vi "201786.vi"() -> ()   [LabVIEW 2013]
doc: "This simple example demonstrates the use of the relative time axis, synchronized with the system clock. This example uses the Timed Loop structure to determine the loop timing as well as the delta X for the points on the strip-chart. \n\nUsing the Timed Loop, along with the correct setting of two of its properties, ensures the accuracy of the time values displayed on the bottom of the chart. Double-click the Input Node of the Timed Loop, to observe the Discard missed periods option is not checked and the Maintain original phase option is checked. If you control timing using the Wait Until Next ms Multiple function, as demonstrated in the example program entitled \"Real-Time Chart\" (refer to the Developer Zone for this example), jitter causes delays in the execution of the While Loop. Over time, these delays complie and the time values displayed at the bottom of the chart drifts from the actual system clock. By using the Timed Loop, you can compensate for unexpected delays in subsequent iterations of the loop. This ensures the time values displayed on the bottom of the chart stay synchronized with the system clock.\n\nYou can use this example as a prototype for applications that acquire data at a constant, known rate. You determine the maximum rate using the timer resolution and speed of your machine. \n\nNote: The Period of Loop (ms) input in this example allows a minimum of 50 ms. This prevents the user from attempting to set the period to less than the actual time needed to execute the iteration. You can change this minimum value by changing the properties of the Period of Loop (ms) input.\n\nNote the use of Unbundle by Name function to extract the current time information, as well as the use of the Chart Property Node to set the X axis as desired. The current example displays 10 seconds of data regardless of the sample rate determined by the Period of Loop (ms) input."
uses:
  <vilib>/Platform/TimedLoop/XDataNode/timing_clust.ctl
  <vilib>/Platform/TimedLoop/XDataNode/nitl_modes.ctl
  <vilib>/Platform/TimedLoop/XDataNode/wakeup.ctl
  <vilib>/platform/TimedLoop/XDataNode/XDataNode.xnode
  <vilib>/Platform/TimedLoop/XDataNode/XDNodeRunTimeDep.lvlib
panel:
  in  "stop":bool
  out "Strip Chart":cluster{dbl, dbl}(graph)={0.6048539044559809, 0.9356575577636529}
  in  "Period of Loop (ms)":u32(knob)=50 min=50 scale=0.0..2000.0
  # "Select Help»Show Context Help and move the cursor\nover the VI icon to display help for this VI."
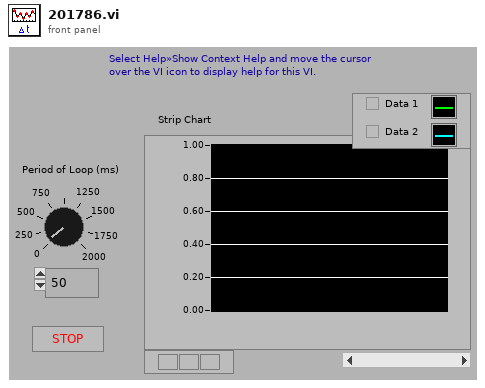
[diagram p1: front panel]
types:
  T1 = cluster{"second":i32, "minute":i32, "hour":i32, "day of month":i32, "month":i32, "year":i32, "day of week":i32, "day of year":i32, "is DST":i32}
  T2 = typedef "XDNodeRunTimeDep.lvlib/timing_clust.ctl" = cluster{"Expected End [f-1]":u64, "Actual End [f-1]":u64, "Finished Late? [f-1]":bool, "Expected End [i-1]":u64, "Actual End [i-1]":u64, "Finished Late? [i-1]":bool, "Expected Start [i]":u64, "Actual Start [i]":u64, "Expected Start [f]":u64, "Actual Start [f]":u64, "Source Name":string, "Structure Name":string, "Period":i64, "Deadline":i64, "Offset":i64, "Start":i64, "Priority":i32, "Timeout":i32, "Mode":T3, "Wakeup Reason":T4, "Error":errorcluster, "Source Type":string, "Secondary Source Type":string, "Global End Time":u64, "Global Start Time":u64, "Frame Duration":u64, "Iteration Duration":u64, "Assigned CPU":i32, "I/O Scan Engine Mode":u32}
  T3 = typedef "XDNodeRunTimeDep.lvlib/nitl_modes.ctl" = enum32{"No Change", "Process missed periods, maintain original phase", "Discard missed periods, maintain original phase", "Process missed periods, ignore original phase", "Discard missed periods, ignore original phase"}
  T4 = typedef "XDNodeRunTimeDep.lvlib/wakeup.ctl" = enum32{"Normal", "Aborted", "Asynchronous wakeup", "Timing source error", "Timed loop error", "Timeout"}
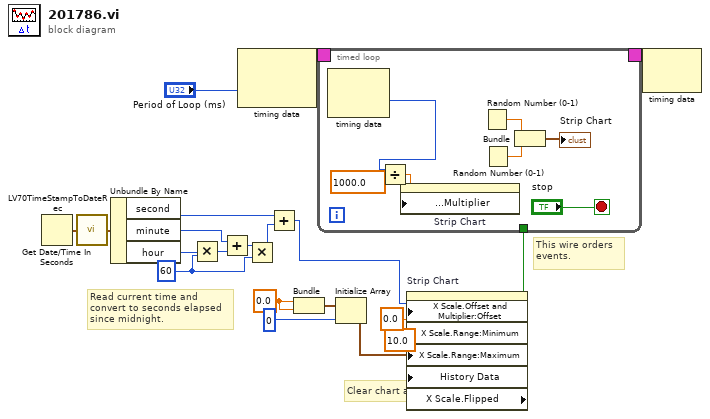
[diagram p0: block diagram]
diagram:
  w9 = 0.0
  w13 = 60
  # "This wire orders\nevents."
  # "Clear chart and set the X axis."
  # "Read current time and\nconvert to seconds elapsed\nsince midnight."
  n1 = Get Date/Time In Seconds() -> (seconds since 1Jan1904=w1:timestamp)
  n2 = call <vilib>:"LV70TimeStampToDateRec.vi"("time stamp"=w1) -> ("date time rec"=w20:T1)
  n3 = Unbundle By Name(w20) -> ("second"=w14:i32, "minute"=w17:i32, "hour"=w19:i32)
  n4 = Multiply(x=w19, y=w13) -> (x*y=w18:i32)
  n5 = Add(x=w17, y=w18) -> (x+y=w16:i32)
  n6 = node-c288("Period of Loop (ms)") -> (w2:T2)  [unwired: 1 in]
  n7 = Multiply(x=w16, y=w13) -> (x*y=w15:i32)
  n8 = Add(x=w14, y=w15) -> (x+y=w5:i32)
  n9 = Bundle(w9, w9) -> (w8:cluster{dbl, dbl})  [unwired: 1 in]
  n10 = Initialize Array(w8, 0) -> (w12:cluster{dbl, dbl}[])
  n11 = property on="Strip Chart" class="WFChart (strict)"("X Scale.Offset and Multiplier:Offset"=w5, "X Scale.Range:Minimum"=0.0, "X Scale.Range:Maximum"=10.0, "History Data"=w12) -> ("X Scale.Flipped"=w10:bool)  [unwired: 2 in, 2 out]
  n12 = timed-loop {
    timing-out: [_] -> w3
    timing: w2 -> [_]
    tunnel: w10 -> [_]
    stop <- "stop" stop-if-true
    n13 = node-c288() -> (w21:i64)  [unwired: 1 in, 1 out]
    n14 = Divide(x=w21, y=1000.0) -> (x/y=w23:dbl)
    n15 = property on="Strip Chart" class="WFChart (strict)"("X Scale.Offset and Multiplier:Multiplier"=w23) -> ()  [unwired: 2 in, 2 out]
    n16 = Random Number (0-1)() -> (number: 0 to 1=w26:dbl)
    n17 = Random Number (0-1)() -> (number: 0 to 1=w27:dbl)
    n18 = Bundle(w26, w27) -> (→"Strip Chart":cluster{dbl, dbl})  [unwired: 1 in]
  }
  n19 = node-c288(w3) -> ()  [unwired: 1 out]
